vi "LIA Test SineCosine Host.vi"() -> ()   [LabVIEW 2017]
uses:
  <vilib>/userdefined/Silver/nirio_resource_slv.ctl
  <vilib>/Analysis/4window.llb/windowTd.ctl
  <vilib>/FPGAPlugInAG/PXIe-7976R/niLvFpga_Open_PXIe-7976R.vi
  <vilib>/rvi/interface/common/dynamic/niFpgaDynamicAddResources.vi
  <vilib>/measure/maspectr.llb/FFT Power Spectrum and PSD for 1 Chan.vi
  <vilib>/Utility/error.llb/Error Cluster From Error Code.vi
  <vilib>/rvi/errors/niLvFpgaAdjustHostInterfaceError.vi
  <vilib>/rvi/interface/common/niFpgaWaitOnOcc.vi
  <instrlib>/_niInstr/Streaming/v1/Host/Public/Start Continuous Stream.vi
  <vilib>/FPGAPlugInAG/Dynamic/niLvFpga_Close_Dynamic.vi
  <vilib>/rvi/interface/nirviOpenFPGA/nirviOpenFPGA.xnode
  FPGA Bitfiles/LIA Basic SineCosine.lvbitx
  <vilib>/rvi/interface/nirviReadWriteControl/nirviReadWriteControl.xnode
  <vilib>/rvi/interface/nirviMethod/nirviMethod.xnode
  <vilib>/ErrorRing/Error Ring.xnode
  <vilib>/rvi/interface/nirviCloseFPGA/nirviCloseFPGA.xnode
  <instrlib>/_niInstr/Streaming/v1/Host/niInstr Streaming v1 Host.lvlib
  <vilib>/rvi/errors/niLvFpgaMergeErrorWithErrorCode.vi
  <vilib>/rvi/interface/Simulation/niFpgaSimulationCallBeginRW.vi
  <vilib>/measure/NI_MAPro.lvlib
  <vilib>/Analysis/NI_AALPro.lvlib
  NiFpgaLv.dll
  <vilib>/FPGAPlugInAG/Dynamic/niLvFpga_StopFifo_Dynamic.vi
  <vilib>/FPGAPlugInAG/Dynamic/niLvFpga_ConfigureFifo_Dynamic.vi
  <vilib>/FPGAPlugInAG/Dynamic/niLvFpga_StartFifo_Dynamic.vi
  <vilib>/FPGAPlugInAG/Dynamic/niLvFpga_ReadFifo_Dynamic.vi
  <vilib>/Analysis/0measdsp.llb/Scaled Time Domain Window (DBL).vi
  <vilib>/Analysis/2dsp.llb/Real FFT.vi
panel:
  out "FIFO rdi count":u64
  out "phase delta (pi rad)":fxp<+/-,20,1> format="%.16g"
  out "Records Processed":i32
  out "Records Read":u32
  out "Actual Depth":u32 format="%.0p"
  out "Samples Transferred":u64
  out "Power Specturm Graph":cluster{"f0":dbl, "df":dbl, "magnitude":dbl[]}(graph)
  in  "Frequency (Hz)":dbl=1000000.0 format="%#_p"
  in  "Sampling Rate (Hz)":dbl=100000000.0 format="%#_p"
  out "Waveform Graph IQ":dbl[][](graph)
  in  "Number of Elements":u32=10000
  in  "Stop Button":bool
  out "error out":errorcluster
  in  "error in":errorcluster
  in  "Resource Name":T1="PXI2Slot2"
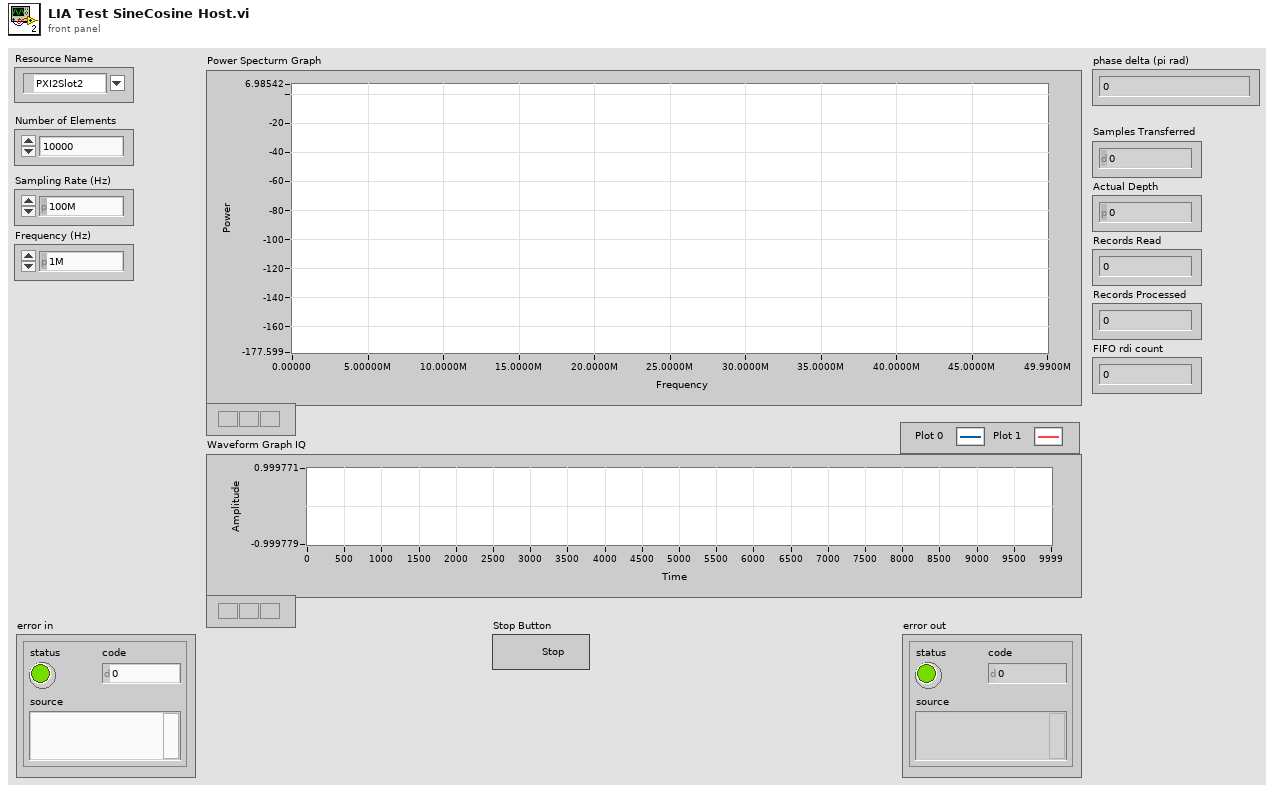
[diagram p1: front panel]
types:
  T1 = typedef "nirio_resource_slv.ctl" = tag
  T2 = typedef "NI_AALPro.lvlib/windowTd.ctl" = u32
  T3 = typedef "niInstr Streaming v1 Common.lvlib/Stream State.ctl" = enum8{"Idle", "Finite Transfer", "Continuous", "Done", "Error", "Not Ready", "Cancel"}
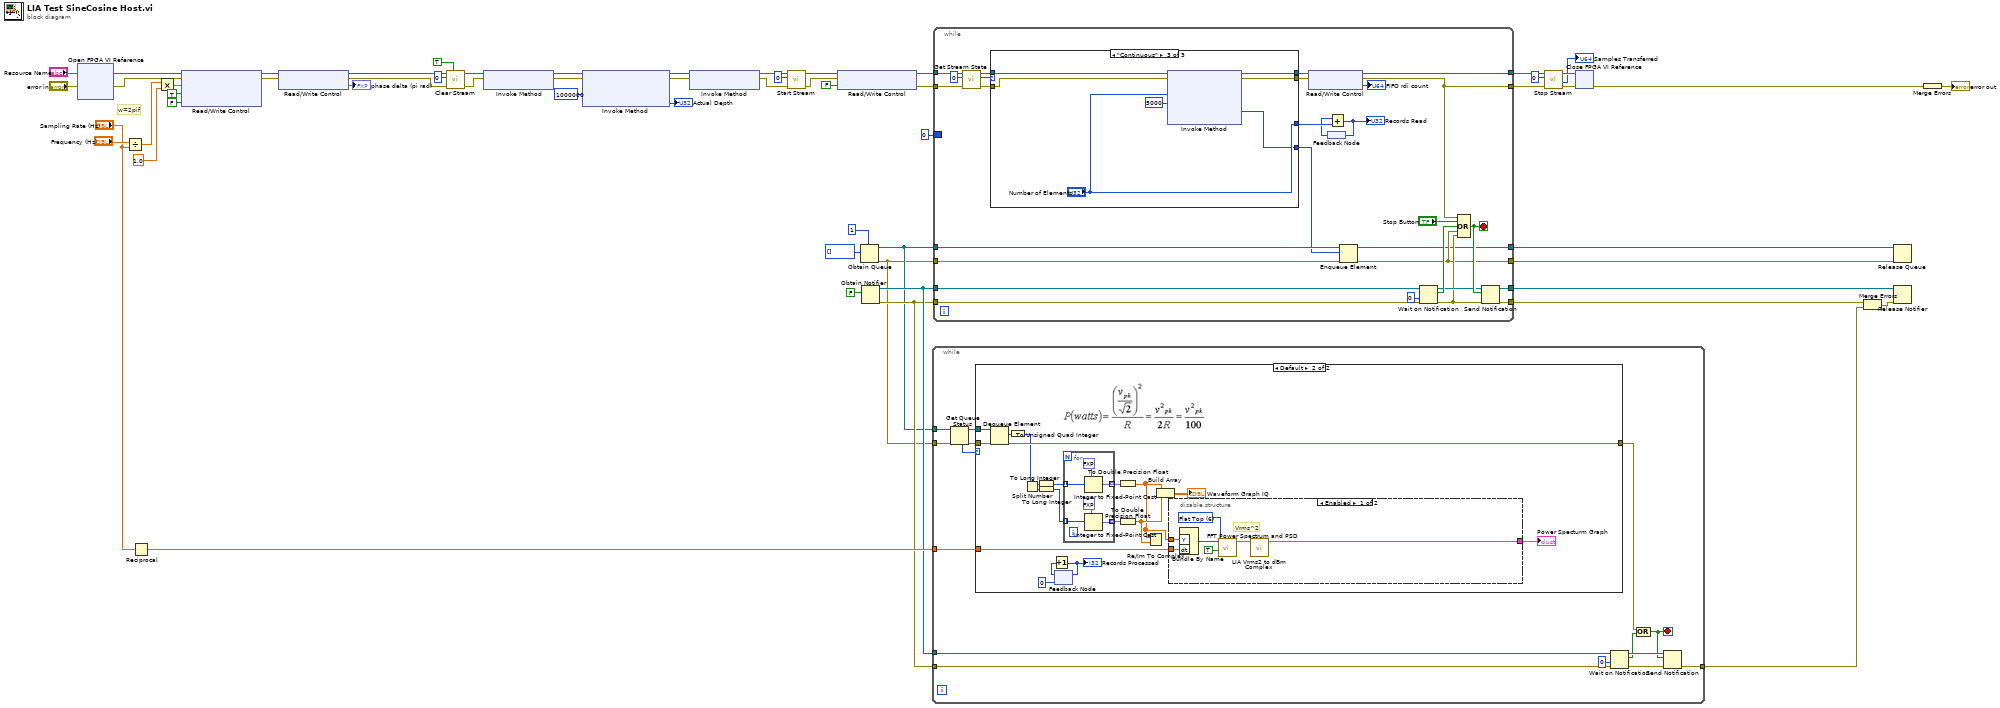
[diagram p0: block diagram]
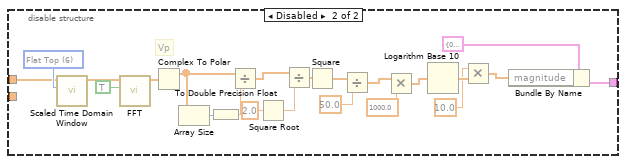
[diagram p3: hidden frame]
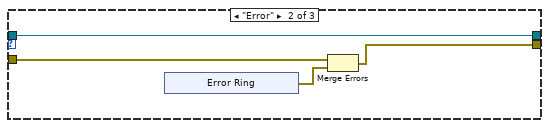
[diagram p5: hidden frame]
diagram:
  # "w=2pif"
  n1 = xnode "Open FPGA VI Reference"("error in"="error in", "resource name"="Resource Name") -> ("FPGA VI Reference Out"=w40:refnum<k20>, "error out"=w55:errorcluster)
  n2 = Divide(x="Frequency (Hz)", y="Sampling Rate (Hz)") -> (x/y=w2:dbl)
  n3 = Reciprocal(x="Sampling Rate (Hz)") -> (1/x=w24:dbl)
  n4 = Multiply(x=w2, y=1.0) -> (x*y=w4:dbl)
  n5 = xnode "Read/Write Control"("FPGA VI Reference In"=w40, "error in"=w55, "phase delta (pi rad)"=w4, "clear rdi counters (T) 0"=TRUE ("reset (T) 0"), "fs?"=FALSE) -> ("FPGA VI Reference Out"=w39:refnum<k20>, "error out"=w38:errorcluster)
  n6 = xnode "Read/Write Control"("FPGA VI Reference In"=w39, "error in"=w38) -> ("FPGA VI Reference Out"=w37:refnum<k20>, "error out"=w36:errorcluster, "phase delta (pi rad)"=→"phase delta (pi rad)":fxp<+/-,20,1>)
  n7 = call <instrlib>:"Clear Stream.vi"("clear on error in?"=TRUE, "error in (no error)"=w36, "stream index"=0, "refnum in"=w37) -> ("error out"=w54:errorcluster, "refnum out"=w50:refnum<k20>)  [unwired: 6 in]
  n8 = xnode "Invoke Method"("FPGA VI Reference In"=w50, "error in"=w54) -> ("FPGA VI Reference Out"=w34:refnum<k20>, "error out"=w51:errorcluster)
  n9 = xnode "Invoke Method"("FPGA VI Reference In"=w34, "error in"=w51, "Requested Depth"=u32 1000000) -> ("FPGA VI Reference Out"=w33:refnum<k20>, "error out"=w35:errorcluster, "Actual Depth"=→"Actual Depth":u32)
  n10 = xnode "Invoke Method"("FPGA VI Reference In"=w33, "error in"=w35) -> ("FPGA VI Reference Out"=w48:refnum<k20>, "error out"=w49:errorcluster)
  n11 = call-poly <instrlib>:"Start Stream.vi"("error in (no error)"=w49, "stream index"=0, "refnum in"=w48) -> ("error out"=w46:errorcluster, "refnum out"=w43:refnum<k20>)  [unwired: 7 in]
  n12 = xnode "Read/Write Control"("FPGA VI Reference In"=w43, "error in"=w46, "clear rdi counters (T) 0"=FALSE ("reset")) -> ("FPGA VI Reference Out"=w42:refnum<k20>, "error out"=w44:errorcluster)
  n13 = Obtain Queue(max queue size (-1, unlimited)=1, element data type=u64[] [] ("Data")) -> (queue out=w12:refnum<queue>, error out=w11:errorcluster)  [unwired: 3 in, 1 out]
  n14 = Obtain Notifier(notification data type=FALSE) -> (notifier out=w18:refnum<notifier>, error out=w17:errorcluster)  [unwired: 3 in, 1 out]
  n15 = while {
    tunnel: w24 -> [w72]
    tunnel: [w66] -> w19
    tunnel: w18 -> [w65]
    tunnel: w17 -> [w64]
    tunnel: w12 -> [w61]
    tunnel: w11 -> [w63]
    stop <- w67 stop-if-true
    n16 = Get Queue Status(queue=w61, error in (no error)=w63) -> (queue out=w60:refnum<queue>, error out=w62:errorcluster, # elements in queue=w59:i32)  [unwired: 1 in, 5 out]
    n17 = case shown="Default" w59 {
      tunnel: w72 -> [_ w92]
      tunnel: w62 -> [w73 w90]
      tunnel: w60 -> [_ w89]
      tunnel: [w73 w88] -> w58
      frame 0 {
      }
      frame Default {
        n18 = Dequeue Element(queue=w89, error in (no error)=w90) -> (element=w91:u64[], error out=w88:errorcluster)  [unwired: 1 in, 2 out]
        n19 = To Unsigned Quad Integer(1:w91) -> (0:w75:u64[])
        n20 = Split Number(x=w75) -> (hi(x)=w85:u32[], lo(x)=w84:u32[])
        n21 = To Long Integer(number=w85) -> (32bit integer=w77:i32[])
        n22 = To Long Integer(number=w84) -> (32bit integer=w76:i32[])
        n23 = feedback #1(0) -> (w86:i32)
        n24 = Increment(x=w86) -> (x+1=w87:i32)
        "Records Processed" <- w87
        n25 = feedback-in #1(w87) -> ()
        n26 = for {
          tunnel: w77 -> [w127] mode=indexing
          tunnel: w76 -> [w126] mode=indexing
          tunnel: [w125] -> w83 mode=indexing
          tunnel: [w124] -> w82 mode=indexing
          n27 = Integer to Fixed-Point Cast(fixed-point type=fxp<+/-,20,2> 0.0, integer=w127) -> (fixed-point=w125:fxp<+/-,20,2>)
          n28 = Integer to Fixed-Point Cast(fixed-point type=fxp<+/-,20,2> 0.0, integer=w126) -> (fixed-point=w124:fxp<+/-,20,2>)
        }
        n29 = To Double Precision Float(number=w83) -> (double precision float=w74:dbl[])
        n30 = To Double Precision Float(number=w82) -> (double precision float=w80:dbl[])
        n31 = Re/Im To Complex(1:w80, 2:w74) -> ()  [unwired: 1 out]
        n32 = Build Array(w74, w80) -> (→"Waveform Graph IQ":dbl[][])
        n33 = disable-structure shown="Enabled" {
          disable-tunnel: w92 -> [w99 _]
          disable-tunnel: w74 -> [w98 w107]
          disable-tunnel: [w94 w101] -> w78
          frame Enabled {
            w93 = T2 6 items=["Rectangle"=0, "Hanning"=1, "Hamming"=2, "Blackman-Harris"=3, "Exact Blackman"=4, "Blackman"=5, "Flat Top"=6, "4 Term B-Harris "=7, "7 Term B-Harris"=8, "Low Sidelobe"=9, "Blackman Nuttall"=11, "Triangle"=30, "Bartlett-Hanning"=31, "Bohman"=32, "Parzen"=33, "Welch"=34, "Kaiser"=60, "Dolph-Chebyshev"=61, "Gaussian"=62] ("window")
            # "Vrms^2"
            n34 = Bundle By Name("Y"=w98, "dt"=w99) -> (w97:waveform(dbl))  [unwired: 1 in]
            n35 = call-poly <vilib>:"FFT Power Spectrum and PSD.vi"("dB On (F)"=TRUE, "window"=w93, "time signal"=w97) -> ("Power Spectrum / PSD"=w95:cluster{"f0":dbl, "df":dbl, "magnitude":dbl[]})  [unwired: 5 in, 3 out]
            n36 = call "LIA Vrms2 to dBm Complex.vi"("Power Spectrum / PSD"=w95) -> ("Power Spectrum / PSD (dBm)"=w94:cluster{"f0":dbl, "df":dbl, "magnitude":dbl[]})  [unwired: 9 in, 1 out]
          }
          frame Disabled {
            w108 = T2 6 items=["Rectangle"=0, "Hanning"=1, "Hamming"=2, "Blackman-Harris"=3, "Exact Blackman"=4, "Blackman"=5, "Flat Top"=6, "4 Term B-Harris "=7, "7 Term B-Harris"=8, "Low Sidelobe"=9, "Blackman Nuttall"=11, "Triangle"=30, "Bartlett-Hanning"=31, "Bohman"=32, "Parzen"=33, "Welch"=34, "Kaiser"=60, "Dolph-Chebyshev"=61, "Gaussian"=62] ("window")
            # "Vp"
            n37 = call-poly <vilib>:"Scaled Time Domain Window.vi"("window"=w108, "X"=w107) -> ("Windowed X"=w106:dbl[])  [unwired: 7 in, 2 out]
            n38 = call-poly <vilib>:"FFT.vi"("shift?"=TRUE, "X"=w106) -> ("FFT {X}"=w121:cdb[])  [unwired: 8 in, 1 out]
            n39 = Complex To Polar(r * e^(i*theta)=w121) -> (r=w120:dbl[])  [unwired: 1 out]
            n40 = Array Size(array=w120) -> (size(s)=w119:i32)
            n41 = To Double Precision Float(number=w119) -> (double precision float=w112:dbl)
            n42 = Divide(x=w120, y=w112) -> (x/y=w105:dbl[])
            n43 = Square Root(x=2.0) -> (sqrt(x)=w110:dbl)
            n44 = Divide(x=w105, y=w110) -> (x/y=w109:dbl[])
            n45 = Square(x=w109) -> (x^2=w104:dbl[])
            n46 = Divide(x=w104, y=50.0) -> (x/y=w115:dbl[])
            n47 = Multiply(x=w115, y=1000.0) -> (x*y=w103:dbl[])
            n48 = Logarithm Base 10(1:w103) -> (0:w117:dbl[])
            n49 = Multiply(x=10.0, y=w117) -> (x*y=w100:dbl[])
            n50 = Bundle By Name(cluster=cluster{"f0":dbl, "df":dbl, "magnitude":dbl[]} {"f0"=0.0, "df"=1.0, "magnitude"=[]} ("Power Spectrum / PSD"), "magnitude"=w100) -> (w101:cluster{"f0":dbl, "df":dbl, "magnitude":dbl[]})
          }
        }
        "Power Specturm Graph" <- w78
      }
    }
    n51 = Wait on Notification(notifier=w65, timeout in ms (-1)=0, error in (no error)=w64) -> (notifier out=w70:refnum<notifier>, notification=w68:bool, error out=w71:errorcluster)  [unwired: 1 in, 1 out]
    n52 = Compound Arithmetic op=OR(w58, w68) -> (w67:bool)
    n53 = Send Notification(notification=w67, notifier=w70, error in (no error)=w71) -> (error out=w66:errorcluster)  [unwired: 1 out]
  }
  n54 = while {
    tunnel: [w129] -> w30
    tunnel: w42 -> [w154]
    tunnel: [w131] -> w31
    tunnel: w44 -> [w152]
    tunnel: [w147] -> w22
    tunnel: w18 -> [w145]
    tunnel: [w148] -> w21
    tunnel: w17 -> [w144]
    tunnel: [w136] -> w14
    tunnel: w12 -> [w137]
    tunnel: [w138] -> w13
    tunnel: w11 -> [w140]
    border: u32 0 -> [_]
    stop <- w146 stop-if-true
    n55 = call <instrlib>:"Get Stream State.vi"("error in (no error)"=w152, "stream index"=0, "refnum in"=w154) -> ("error out"=w151:errorcluster, "stream state"=w150:T3, "refnum out"=w153:refnum<k20>)  [unwired: 6 in]
    n56 = case shown="\"Continuous\"" w150 {
      tunnel: [w157 w160 w173] -> w156
      tunnel: [w158 w162 w172] -> w130
      tunnel: w153 -> [w158 w162 w171]
      tunnel: w151 -> [w157 w161 w170]
      tunnel: [_ _ w169] -> w135
      tunnel: [_ _ "Number of Elements"] -> w134
      frame Default {
      }
      frame "Error" {
        n57 = xnode "Error Ring"() -> ("error out"=w159:errorcluster)
        n58 = Merge Errors(w161, w159) -> (w160:errorcluster)
      }
      frame "Continuous" {
        n59 = xnode "Invoke Method"("FPGA VI Reference In"=w171, "error in"=w170, "Number of Elements"="Number of Elements", "Timeout (ms)"=5000) -> ("FPGA VI Reference Out"=w172:refnum<k20>, "error out"=w173:errorcluster, "Data"=w169:u64[])  [unwired: 1 out]
      }
    }
    n60 = xnode "Read/Write Control"("FPGA VI Reference In"=w130, "error in"=w156) -> ("FPGA VI Reference Out"=w129:refnum<k20>, "error out"=w131:errorcluster, "FIFO rdi count"=→"FIFO rdi count":u64)
    n61 = feedback #2() -> (w133:u32)
    n62 = Add(x=w133, y=w134) -> (x+y=w132:u32)
    "Records Read" <- w132
    n63 = feedback-in #2(w132) -> ()
    n64 = Enqueue Element(queue=w137, element=w135, error in (no error)=w140) -> (queue out=w136:refnum<queue>, error out=w138:errorcluster)  [unwired: 1 in, 1 out]
    n65 = Wait on Notification(notifier=w145, timeout in ms (-1)=0, error in (no error)=w144) -> (notifier out=w141:refnum<notifier>, notification=w142:bool, error out=w139:errorcluster)  [unwired: 1 in, 1 out]
    n66 = Compound Arithmetic op=OR(w131, "Stop Button", w142, w138, w139) -> (w146:bool)
    n67 = Send Notification(notification=w146, notifier=w141, error in (no error)=w139) -> (notifier out=w147:refnum<notifier>, error out=w148:errorcluster)
  }
  n68 = call <instrlib>:"Stop Stream.vi"("error in (no error)"=w31, "stream index"=0, "refnum in"=w30) -> ("error out"=w28:errorcluster, "samples transferred"=→"Samples Transferred":u64, "refnum out"=w29:refnum<k20>)  [unwired: 5 in, 1 out]
  n69 = xnode "Close FPGA VI Reference"("FPGA VI Reference In"=w29, "error in"=w28) -> ("error out"=w45:errorcluster)
  n70 = Merge Errors(w21, w19) -> (w20:errorcluster)
  n71 = Release Queue(queue=w14, error in (no error)=w13) -> ()  [unwired: 1 in, 3 out]
  n72 = Release Notifier(notifier=w22, error in (no error)=w20) -> ()  [unwired: 1 in, 3 out]
  n73 = Merge Errors(w45) -> (→"error out":errorcluster)
